vi "Generate write queue item.vi"(8 "error in (no error)":errorcluster, 10 "Request ID":u64, 11 "wamplv.lvlib:CallRequest (JSON).lvclass":refnum<class "CallRequest (JSON).lvclass">) -> (0 "error out":errorcluster, 3 "Write queue item":T1)   [LabVIEW 2020, in "wamplv.lvlib" / "CallRequest (JSON).lvclass"]
uses:
  CallRequest (JSON).lvclass
  CallRequest (JSON).lvclass/CallRequest (JSON).ctl
  TypeDefs/WAMP Message Codes.ctl
  wamplv.lvlib
  Utils/Utils.lvclass
  8d3f56c2-5707-484f-8241-7d0afc6948b6.vi
  TypeDefs/Transport type.ctl
  WAMP Client/Private/TypeDef/Write queue item.ctl
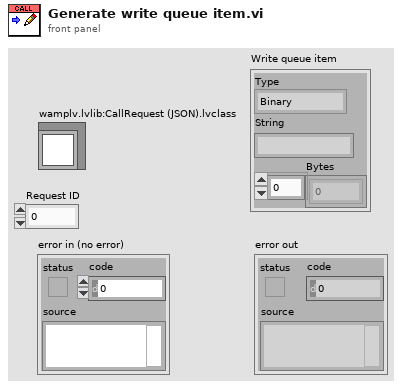
[diagram p1: front panel]
types:
  T1 = typedef "wamplv.lvlib/Write queue item.ctl" = cluster{"Type":T2, "String":string, "Bytes":u8[]}
  T2 = typedef "wamplv.lvlib/Transport type.ctl" = enum16{"Binary", "Text"}
  T3 = typedef "wamplv.lvlib/WAMP Message Codes.ctl" = u16
  T4 = typedef "wamplv.lvlib/CALL request (JSON).ctl" = cluster{"Topic URI":string, "Arguments":string, "ArgumentsKw":string, "Options":string, "Call result":refnum<notifier>}
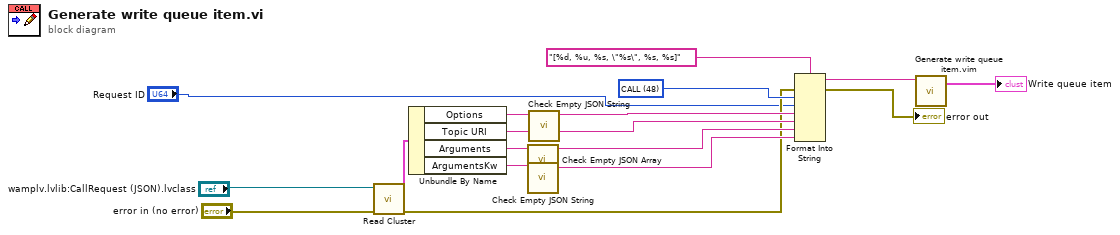
[diagram p0: block diagram]
diagram:
  w9 = T3 48 items=["HELLO"=1, "WELCOME"=2, "ABORT"=3, "GOODBYE"=6, "ERROR"=8, "PUBLISH"=16, "PUBLISHED"=17, "SUBSCRIBE"=32, "SUBSCRIBED"=33, "UNSUBSCRIBE"=34, "UNSUBSCRIBED"=35, "EVENT"=36, "CALL"=48, "RESULT"=59, "REGISTER"=64, "REGISTERED"=65, "UNREGISTER"=66, "UNREGISTERED"=67, "INVOCATION"=68, "YIELD"=70] ("Message Codes")
  n1 = call "Read Cluster.vi"("error in (no error)"="error in (no error)", "CallRequest (JSON) in"="wamplv.lvlib:CallRequest (JSON).lvclass") -> ("error out"=w7:errorcluster, "Cluster"=w8:T4)  [unwired: 7 in, 1 out]
  n2 = Unbundle By Name(w8) -> ("Options"=w12:string, "Topic URI"=w15:string, "Arguments"=w16:string, "ArgumentsKw"=w14:string)
  n3 = call "Check Empty JSON Array.vi"("JSON in"=w16) -> ("JSON out"=w17:string)  [unwired: 10 in]
  n4 = call "Check Empty JSON String.vi"("JSON in"=w14) -> ("JSON out"=w13:string)  [unwired: 10 in]
  n5 = call "Check Empty JSON String.vi"("JSON in"=w12) -> ("JSON out"=w11:string)  [unwired: 10 in]
  n6 = Format Into String(format string="[%d, %u, %s, \"%s\", %s, %s]" ("element"), error in=w7, w9, "Request ID", w11, w15, w17, w13) -> (resulting string=w3:string, error out=→"error out":errorcluster)  [unwired: 1 in]
  n7 = call "Generate write queue item.vim"("Input"=w3) -> ("Ouput"=→"Write queue item":T1)  [unwired: 2 in]
